vi "Position Adding.vi"(11 "System":string="3") -> ()   [LabVIEW 2023]
uses:
  <vilib>/Utility/file.llb/Read Delimited Spreadsheet (I64).vi
  <vilib>/Utility/file.llb/Read Delimited Spreadsheet (string).vi
  <vilib>/Utility/file.llb/Write Delimited Spreadsheet (string).vi
panel:
  in  "Exit":bool
  out "Message":string
  in  "Rack Number":i32=1 min=1 max=16 step=1
  out "Unit_Number(out)":string="XXXXXXXXXXX"
  out "Work Order(out)":string="XXXXX-XXX"
  in  "Unit_Number":string
  in  "Work Order":string
  out "Rack Number(out)":i32=2 min=2 max=15
  out "Number of Units(out)":i32 min=1 max=32 step=1
  in  "Enter":bool
  in  "Number of Units":i32=1 min=1 max=40 step=1
  out "Serial Numbers":string[](array[string])
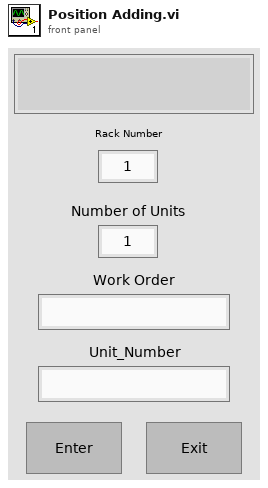
[diagram p1: front panel]
types:
  T1 = enum16{"open", "replace", "create", "open or create", "replace or create", "replace or create with confirmation"}
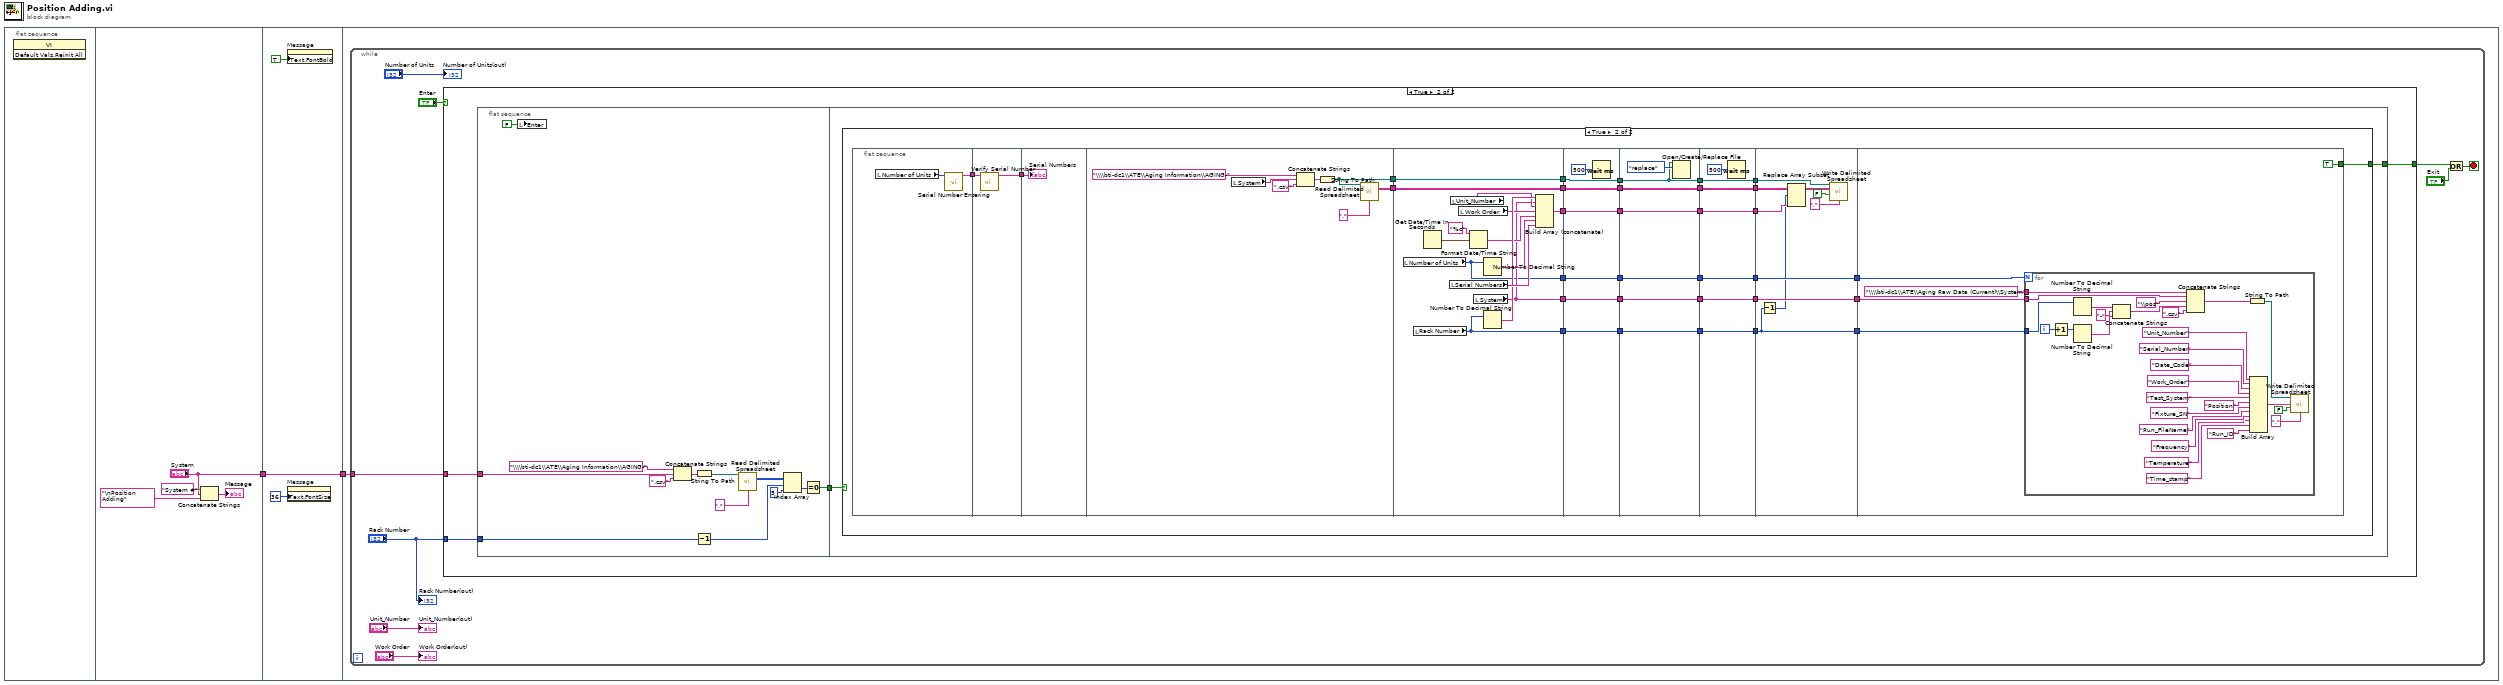
[diagram p0: block diagram]
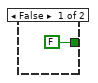
[diagram p2: hidden frame]
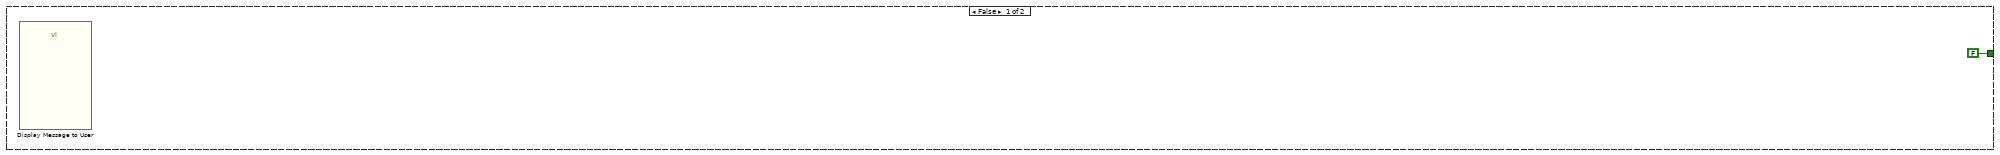
[diagram p3: hidden frame]
diagram:
  n1 = flat-sequence {
    tunnel: ["System"] -> w1
    tunnel: [w7] -> w2
    tunnel: w1 -> [w7]
    tunnel: w2 -> [w10]
    frame #0 {
      n2 = invoke class="VI" method="Default Vals.Reinit All"() -> ()  [unwired: 3 in, 3 out]
    }
    frame #1 {
      n3 = Concatenate Strings("System #" ("Message"), "System", "\nPosition Adding" ("string")) -> (→"Message":string)
    }
    frame #2 {
      n4 = property on="Message" class="Str"("Text.FontBold"=TRUE ("Text.Font:Bold")) -> ()  [unwired: 2 in, 2 out]
      n5 = property on="Message" class="Str"("Text.FontSize"=u32 36 ("Text.Font:Size")) -> ()  [unwired: 2 in, 2 out]
    }
    frame #3 {
      n6 = while {
        tunnel: w10 -> [w11]
        stop <- w13 stop-if-true
        n7 = case shown="True" "Enter" {
          tunnel: [FALSE w24] -> w15
          tunnel: "Rack Number" -> [_ w22]
          tunnel: w11 -> [_ w21]
          frame False {
          }
          frame True {
            n8 = flat-sequence {
              tunnel: [w25] -> w23
              tunnel: w22 -> [w28]
              tunnel: w21 -> [w34]
              tunnel: [w39] -> w24
              tunnel: w23 -> [w38]
              frame #0 {
                n9 = local write "Enter"(FALSE ("Enter")) -> ()
                n10 = Concatenate Strings("\\\\bti-dc1\\ATE\\Aging Information\\AGING-" ("string"), w34, ".csv" ("string")) -> (w33:string)
                n11 = String To Path(string=w33) -> (path=w32:path)
                n12 = Decrement(x=w28) -> (x-1=w27:i32)
                n13 = call-poly <vilib>:"Read Delimited Spreadsheet.vi"("file path (dialog if empty)"=w32, "delimiter (\\t)"="," ("delimiter (\\t)")) -> ("all rows"=w30:i64[][])  [unwired: 8 in, 5 out]
                n14 = Index Array(array=w30, index (row)=w27, index (col)=5 ("disabled index (col)")) -> (element=w26:i64)
                n15 = Equal To 0?(x=w26) -> (x = 0?=w25:bool)
              }
              frame #1 {
                n16 = case shown="True" w38 {
                  tunnel: [FALSE w72] -> w39
                  frame False {
                    n17 = call "Display Message to User"() -> ()  [unwired: 10 in, 2 out]
                  }
                  frame True {
                    n18 = flat-sequence {
                      tunnel: [w73] -> w71
                      tunnel: w71 -> [w76]
                      tunnel: [w75] -> w70
                      tunnel: w70 -> [w77]
                      tunnel: [w83] -> w69
                      tunnel: [w82] -> w68
                      tunnel: w69 -> [w98]
                      tunnel: [w98] -> w67
                      tunnel: [w97] -> w66
                      tunnel: [w94] -> w65
                      tunnel: w68 -> [w93]
                      tunnel: [w93] -> w64
                      tunnel: [w86] -> w47
                      tunnel: [w85] -> w42
                      tunnel: w67 -> [w105]
                      tunnel: [w105] -> w59
                      tunnel: w66 -> [w104]
                      tunnel: [w104] -> w57
                      tunnel: w65 -> [w103]
                      tunnel: [w103] -> w55
                      tunnel: w64 -> [w102]
                      tunnel: [w102] -> w53
                      tunnel: [w100] -> w48
                      tunnel: w47 -> [w100]
                      tunnel: [w99] -> w43
                      tunnel: w42 -> [w99]
                      tunnel: w59 -> [w112]
                      tunnel: [w112] -> w58
                      tunnel: w57 -> [w111]
                      tunnel: [w111] -> w56
                      tunnel: w55 -> [w110]
                      tunnel: [w110] -> w54
                      tunnel: w53 -> [w108]
                      tunnel: [w108] -> w52
                      tunnel: [w107] -> w49
                      tunnel: w48 -> [w107]
                      tunnel: [w106] -> w44
                      tunnel: w43 -> [w106]
                      tunnel: w58 -> [w119]
                      tunnel: [w119] -> w63
                      tunnel: w56 -> [w118]
                      tunnel: [w118] -> w62
                      tunnel: w54 -> [w117]
                      tunnel: [w117] -> w61
                      tunnel: w52 -> [w116]
                      tunnel: [w116] -> w60
                      tunnel: [w114] -> w50
                      tunnel: w49 -> [w114]
                      tunnel: [w113] -> w45
                      tunnel: w44 -> [w113]
                      tunnel: w63 -> [w129]
                      tunnel: w62 -> [w120]
                      tunnel: w61 -> [w128]
                      tunnel: w60 -> [w126]
                      tunnel: [w123] -> w51
                      tunnel: w50 -> [w123]
                      tunnel: [w122] -> w46
                      tunnel: w45 -> [w122]
                      tunnel: [w120] -> w41
                      tunnel: [TRUE] -> w72
                      tunnel: w51 -> [w132]
                      tunnel: w46 -> [w131]
                      tunnel: w41 -> [w130]
                      frame #0 {
                        n19 = local read "Number of Units"() -> (w74:i32)
                        n20 = call "Serial Number Entering.vi"("Number of Units"=w74) -> ("Serial Numbers"=w73:string[])  [unwired: 10 in]
                      }
                      frame #1 {
                        n21 = call "Verify Serial Number.vi"("Serial Numbers"=w76) -> ("Serial Numbers(out)"=w75:string[])  [unwired: 10 in]
                      }
                      frame #2 {
                        "Serial Numbers" <- w77
                      }
                      frame #3 {
                        n22 = local read "System"() -> (w79:string)
                        n23 = Concatenate Strings("\\\\bti-dc1\\ATE\\Aging Information\\AGING-" ("string"), w79, ".csv" ("string")) -> (w78:string)
                        n24 = String To Path(string=w78) -> (path=w82:path)
                        n25 = call-poly <vilib>:"Read Delimited Spreadsheet.vi"("file path (dialog if empty)"=w82, "delimiter (\\t)"="," ("delimiter (\\t)")) -> ("all rows"=w83:string[][])  [unwired: 8 in, 5 out]
                      }
                      frame #4 {
                        n26 = local read "Number of Units"() -> (w85:i32)
                        n27 = local read "Rack Number"() -> (w97:i32)
                        n28 = Get Date/Time In Seconds() -> (seconds since 1Jan1904=w89:timestamp)
                        n29 = local read "Serial Numbers"() -> (w95:string[])
                        n30 = local read "Unit_Number"() -> (w91:string)
                        n31 = local read "Work Order"() -> (w90:string)
                        n32 = Format Date/Time String(time format string (%c)="%c", seconds (now)=w89) -> (date/time string=w87:string)  [unwired: 1 in]
                        n33 = local read "System"() -> (w86:string)
                        n34 = Number To Decimal String(number=w85) -> (decimal integer string=w96:string)  [unwired: 1 in]
                        n35 = Number To Decimal String(number=w97) -> (decimal integer string=w92:string)  [unwired: 1 in]
                        n36 = Build Array (concatenate)(w92, w86, w91, w90, w87, w96, w95) -> (w94:string[])
                      }
                      frame #5 {
                        n37 = Wait (ms)(milliseconds to wait=u32 500) -> ()  [unwired: 1 out]
                      }
                      frame #6 {
                        n38 = Open/Create/Replace File(file path (use dialog)=w108, operation (0:open)=T1."replace") -> ()  [unwired: 4 in, 3 out]
                      }
                      frame #7 {
                        n39 = Wait (ms)(milliseconds to wait=u32 500) -> ()  [unwired: 1 out]
                      }
                      frame #8 {
                        n40 = Decrement(x=w120) -> (x-1=w121:i32)
                        n41 = Replace Array Subset(array=w129, new element=w128, index (row)=w121) -> (w127:string[][])  [unwired: 1 in]
                        n42 = call-poly <vilib>:"Write Delimited Spreadsheet.vi"("file path (dialog if empty)"=w126, "2D data"=w127, "append to file? (new file:F)"=FALSE, "delimiter (\\t)"="," ("delimiter (\\t)")) -> ()  [unwired: 10 in, 2 out]
                      }
                      frame #9 {
                        n43 = for {
                          N: w131 -> [_]
                          tunnel: "\\\\bti-dc1\\ATE\\Aging Raw Data (Current)\\System" ("string") -> [w143]
                          tunnel: w132 -> [w142]
                          tunnel: w130 -> [w135]
                          i -> [w141]
                          n44 = Increment(x=w141) -> (x+1=w140:i32)
                          n45 = Number To Decimal String(number=w135) -> (decimal integer string=w139:string)  [unwired: 1 in]
                          n46 = Number To Decimal String(number=w140) -> (decimal integer string=w138:string)  [unwired: 1 in]
                          n47 = Concatenate Strings(w139, "-" ("string"), w138) -> (w136:string)
                          n48 = Concatenate Strings(w143, w142, "\\pos" ("string"), w136, ".csv" ("string")) -> (w160:string)
                          n49 = String To Path(string=w160) -> (path=w161:path)
                          n50 = Build Array("Unit_Number" ("string"), "Serial_Number" ("element"), "Date_Code" ("element"), "Work_Order" ("element"), "Test_System" ("element"), "Position" ("element"), "Fixture_SN" ("element"), "Run_FileName" ("element"), "Frequency" ("element"), "Temperature" ("element"), "Time_stamp" ("element"), "Run_ID" ("element")) -> (w162:string[])
                          n51 = call-poly <vilib>:"Write Delimited Spreadsheet.vi"("file path (dialog if empty)"=w161, "1D data"=w162, "append to file? (new file:F)"=FALSE, "delimiter (\\t)"="," ("delimiter (\\t)")) -> ()  [unwired: 10 in, 2 out]
                        }
                      }
                    }
                  }
                }
              }
            }
          }
        }
        n52 = Or(x=w15, y="Exit") -> (x .or. y?=w13:bool)
        "Number of Units(out)" <- "Number of Units"
        "Rack Number(out)" <- "Rack Number"
        "Work Order(out)" <- "Work Order"
        "Unit_Number(out)" <- "Unit_Number"
      }
    }
  }
